vi "BuildCustomDashBoardData.vi"   [LabVIEW 2013]
doc: "This VI builds data and sends it back to the dashboard PC program. By default it sends back the raw values for the first analog, digital, and solenoid module. Modify it to send back the data you want to view. Consider adding higher level data to the Dashboard Datatype.ctl and to this VI. Then update the Dashboard to display the data however you like.\n\nThis software is licensed. Open the labview\\readme\\WPI Robotics Library Open Source License.txt file for more information."
uses:
  <vilib>/Rock Robotics/WPI/DriverStation/WPI_DriverStationDigitalData.ctl
  typedefs/Dashboard Datatype.ctl
  typedefs/DashboardEnable.ctl
  typedefs/custom dash data.ctl
  typedefs/subStates.ctl
  typedefs/vision data.ctl
  <vilib>/Rock Robotics/WPI/Joystick/WPI_JoystickButtonState.ctl
  typedefs/fg_typedef.ctl
  <vilib>/Rock Robotics/SystemInterfaces/System/FPGA_SystemGet.vi
  <vilib>/Rock Robotics/WPI/Joystick/WPI_JoystickGetSetRefNum.vi
  <vilib>/NI_Real-Time Target Support.lvlib
types:
  T1 = typedef "custom dash data.ctl" = cluster{"Motors":cluster{"Pickup Motor":dbl, "Pickup Belt":dbl, "Pickup Distance ":dbl, "Pickup Rate":dbl, "Right Motor":dbl, "Left Motor":dbl}, "substates":cluster{"Latch":T2, "Pickup Arm":T2, "Belts":T2, "Shooter":T2, "Drive":T2}, "Safeties":cluster{"Arm Safety":bool, "Arm Limit":bool}, "Performance":cluster{"CPU Usage":dbl, "Vision mSPI":u32, "Main mSPI":u32}, "Data":T3, "Joysticks":cluster{"J1 Axes":cluster{"axis 1 (x)":dbl, "axis 2 (y)":dbl, "axis 3 (throttle)":dbl, "axis 4":dbl, "axis 5":dbl, "axis 6":dbl}, "J1 Buttons":T4, "J2 Axes":cluster{"axis 1 (x)":dbl, "axis 2 (y)":dbl, "axis 3 (throttle)":dbl, "axis 4":dbl, "axis 5":dbl, "axis 6":dbl}, "J2 Buttons":T4, "J3 Axes":cluster{"axis 1 (x)":dbl, "axis 2 (y)":dbl, "axis 3 (throttle)":dbl, "axis 4":dbl, "axis 5":dbl, "axis 6":dbl}, "J3 Buttons":T4}, "SubSystem Manager":cluster{"Ball State Read":enum16{"no ball", "holding", "loaded"}, "Picked Up":bool, "Loaded":bool, "Shooter Cocked":bool, "Arm Ready":bool}, "Vision Enabled?":bool}
  T2 = typedef "subStates.ctl" = enum16{"null", "wait", "driver control", "auto", "manual override", "hold position", "rotate", "pickup", "pass", "load", "goto shoot", "shoot", "end"}
  T3 = typedef "vision data.ctl" = cluster{"x":dbl, "y":dbl, "area":dbl, "width":dbl, "height":dbl, "Hot Goal Present?":bool, "distance":dbl}
  T4 = typedef "WPI_JoystickButtonState.ctl" = cluster{"Button 1":bool, "Button 2":bool, "Button 3":bool, "Button 4":bool, "Button 5":bool, "Button 6":bool, "Button 7":bool, "Button 8":bool, "Button 9":bool, "Button 10":bool, "Button 11":bool, "Button 12":bool}
  T5 = typedef "DashboardEnable.ctl" = cluster{"Analog Module 1":bool[], "Analog Module 2":bool[], "Digital Module 1":bool, "Digital Module 2":bool, "Solenoid Module":bool}
  T6 = typedef "Dashboard Datatype.ctl" = cluster{cluster{"AnalogModule[0]":cluster{"Channel[0]":sgl, "Channel[1]":sgl, "Channel[2]":sgl, "Channel[3]":sgl, "Channel[4]":sgl, "Channel[5]":sgl, "Channel[6]":sgl, "Channel[7]":sgl}, "AnalogModule[1]":cluster{"Channel[0]":sgl, "Channel[1]":sgl, "Channel[2]":sgl, "Channel[3]":sgl, "Channel[4]":sgl, "Channel[5]":sgl, "Channel[6]":sgl, "Channel[7]":sgl}}, cluster{"DigitalModule[0]":T7, "DigitalModule[1]":T7}, "Solenoid":u8}
  T7 = typedef "WPI_DriverStationDigitalData.ctl" = cluster{"Relay Fwd":u8, "Relay Rev":u8, "GPIO":u16, "GPIO_OE":u16, "PWM":cluster{"PWM[0]":u8, "PWM[1]":u8, "PWM[2]":u8, "PWM[3]":u8, "PWM[4]":u8, "PWM[5]":u8, "PWM[6]":u8, "PWM[7]":u8, "PWM[8]":u8, "PWM[9]":u8}}
  T8 = typedef "fg_typedef.ctl" = enum16{"Get", "Set"}
  T9 = cluster{"AnalogModule[0]":cluster{"Channel[0]":sgl, "Channel[1]":sgl, "Channel[2]":sgl, "Channel[3]":sgl, "Channel[4]":sgl, "Channel[5]":sgl, "Channel[6]":sgl, "Channel[7]":sgl}, "AnalogModule[1]":cluster{"Channel[0]":sgl, "Channel[1]":sgl, "Channel[2]":sgl, "Channel[3]":sgl, "Channel[4]":sgl, "Channel[5]":sgl, "Channel[6]":sgl, "Channel[7]":sgl}}
  T10 = cluster{"DigitalModule[0]":T7, "DigitalModule[1]":T7}
  T11 = cluster{"Channel[0]":sgl, "Channel[1]":sgl, "Channel[2]":sgl, "Channel[3]":sgl, "Channel[4]":sgl, "Channel[5]":sgl, "Channel[6]":sgl, "Channel[7]":sgl}[]
  T12 = cluster{"Channel[0]":sgl, "Channel[1]":sgl, "Channel[2]":sgl, "Channel[3]":sgl, "Channel[4]":sgl, "Channel[5]":sgl, "Channel[6]":sgl, "Channel[7]":sgl}
  T13 = cluster{"AnalogModule[0][0]":sgl, "AnalogModule[0][1]":sgl, "AnalogModule[0][2]":sgl, "AnalogModule[0][3]":sgl, "AnalogModule[0][4]":sgl, "AnalogModule[0][5]":sgl, "AnalogModule[0][6]":sgl, "AnalogModule[0][7]":sgl}
  T14 = cluster{"[0]":cluster{"Channel[0]":sgl, "Channel[1]":sgl, "Channel[2]":sgl, "Channel[3]":sgl, "Channel[4]":sgl, "Channel[5]":sgl, "Channel[6]":sgl, "Channel[7]":sgl}, "[1]":cluster{"Channel[0]":sgl, "Channel[1]":sgl, "Channel[2]":sgl, "Channel[3]":sgl, "Channel[4]":sgl, "Channel[5]":sgl, "Channel[6]":sgl, "Channel[7]":sgl}}
  T15 = typedef "FPGA_DIODevRef.ctl" = cluster{"DevStatus":errorcluster, "Module":T16}
  T16 = typedef "FPGA_TypedefDigitalModule.ctl" = enum16{"Digital Module 1", "Digital Module 2"}
  T17 = cluster{"[0]":u8, "[1]":u8, "[2]":u8, "[3]":u8, "[4]":u8, "[5]":u8, "[6]":u8, "[7]":u8, "[8]":u8, "[9]":u8}
  T18 = typedef "FPGA_SolenoidDevRef.ctl" = cluster{"DevStatus":errorcluster, "Module":T19}
  T19 = typedef "FPGA_TypedefSolenoidModule.ctl" = enum16{"Solenoid Module 1", "Solenoid Module 2"}
  T20 = cluster{"Pickup Motor":dbl, "Pickup Belt":dbl, "Pickup Distance ":dbl, "Pickup Rate":dbl, "Right Motor":dbl, "Left Motor":dbl}
  T21 = cluster{"CPU Usage":dbl, "Vision mSPI":u32, "Main mSPI":u32}
  T22 = typedef "WPI_EncoderDevRef.ctl" = cluster{"DevStatus":errorcluster, "EncoderIndex":T23, "CounterIndex":T24, "DistancePerCount":dbl, "Decoding Type":T25}
  T23 = typedef "FPGA_EncoderIdx.ctl" = enum8{"Enc 0", "Enc 1", "Enc 2", "Enc 3", "Invalid"}
  T24 = typedef "FPGA_CounterCtrSystemIndex.ctl" = enum8{"Ctr 0", "Ctr 1", "Ctr 2", "Ctr 3", "Ctr 4", "Ctr 5", "Ctr 6", "Ctr 7", "Invalid"}
  T25 = typedef "WPI_EncoderType.ctl" = enum16{"1x", "2x", "4x"}
  T26 = typedef "WPI_MotorControlDeviceRef.ctl" = cluster{"DeviceStatus":errorcluster, "Type":enum16{"PWM", "CAN"}, "PWM":cluster{"Digital Module":T16, "PWM Channel":T27, "DeadBand":T28}, "CAN":cluster{"Device Number":u8, "Control Mode":T29, "Semaphore":T30, "Max Vout":dbl}, "Invert":bool, "TransformRef":T31, "InvTransformRef":T31}
  T27 = typedef "FPGA_DIOPWMChannel.ctl" = enum8{"PWM 1", "PWM 2", "PWM 3", "PWM 4", "PWM 5", "PWM 6", "PWM 7", "PWM 8", "PWM 9", "PWM 10", "Invalid"}
  T28 = typedef "WPI_PWMDeadband.ctl" = cluster{"Name":string, "maxPositivePwm":i32, "minPositivePwm":i32, "centerPwm":i32, "maxNegativePwm":i32, "minNegativePwm":i32, "angularRange":u16}
  T29 = typedef "WPI_CANJaguar_ControlMode.ctl" = enum8{"Percent VBus", "Current", "Speed", "Position", "Voltage"}
  T30 = typedef "Semaphore RefNum" = refnum<k1>
  T31 = typedef "WPI_PWMTransform_ConPane.ctl" = refnum<vi>
  T32 = typedef "NI_Real-Time Target Support.lvlib/RT CPU Load.ctl" = cluster{"Total (%)":dbl, "Time Critical (%)":dbl, "Timed Structures (%)":dbl, "High (%)":dbl, "Above Normal (%)":dbl, "Normal (%)":dbl, "Background (%)":dbl, "Idle (%)":dbl, "ISR (%)":dbl}
  T33 = cluster{"Vision mSPI":u32, "Main mSPI":u32, "Dash mSPI":u32}
  T34 = cluster{"Ball State Read":enum16{"no ball", "holding", "loaded"}, "Picked Up":bool, "Loaded":bool, "Shooter Cocked":bool, "Arm Ready":bool}
  T35 = typedef "WPI_JoystickDevRef.ctl" = cluster{"Device":T36}
  T36 = typedef "WPI_JoystickDeviceEnum.ctl" = enum16{"USB 1", "USB 2", "USB 3", "USB 4", "Kinect 1", "Kinect 2"}
  T37 = cluster{"axis 1 (x)":dbl, "axis 2 (y)":dbl, "axis 3 (throttle)":dbl, "axis 4":dbl, "axis 5":dbl, "axis 6":dbl}
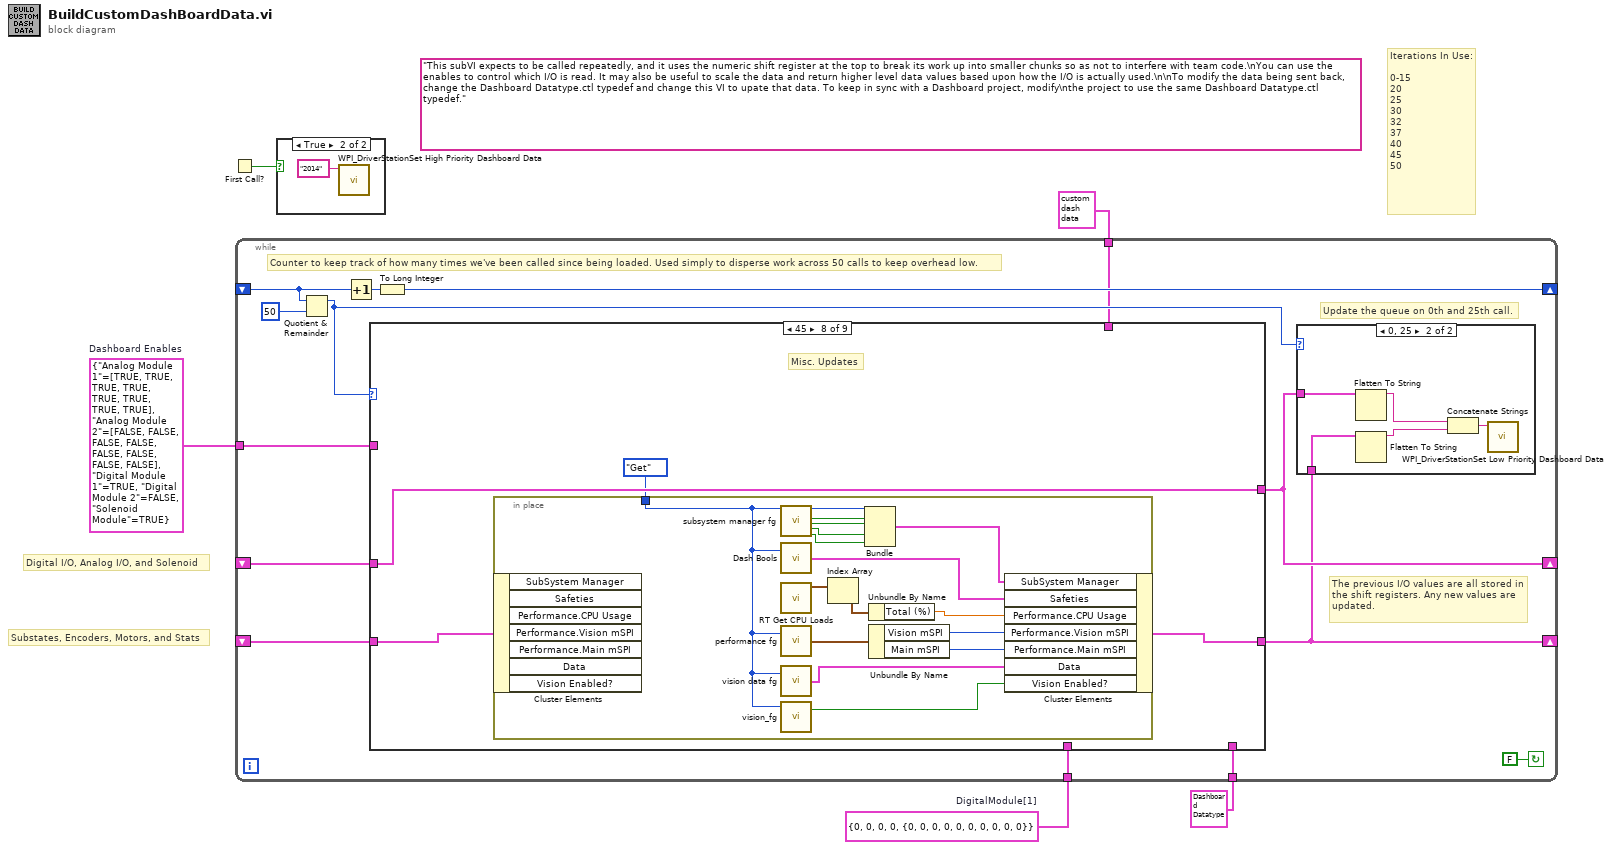
[diagram p0: block diagram]
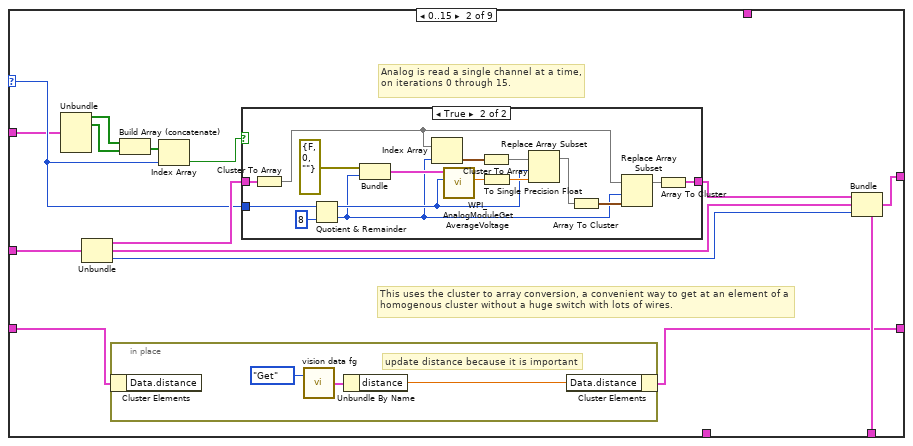
[diagram p5: hidden frame]
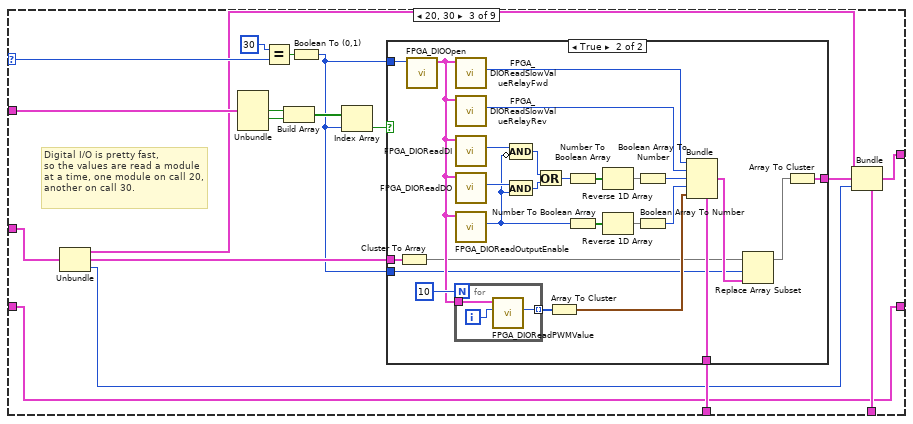
[diagram p7: hidden frame]
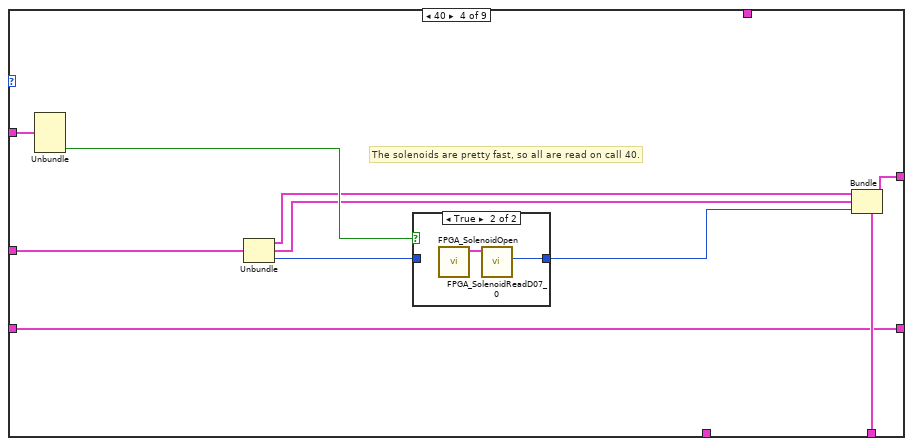
[diagram p9: hidden frame]
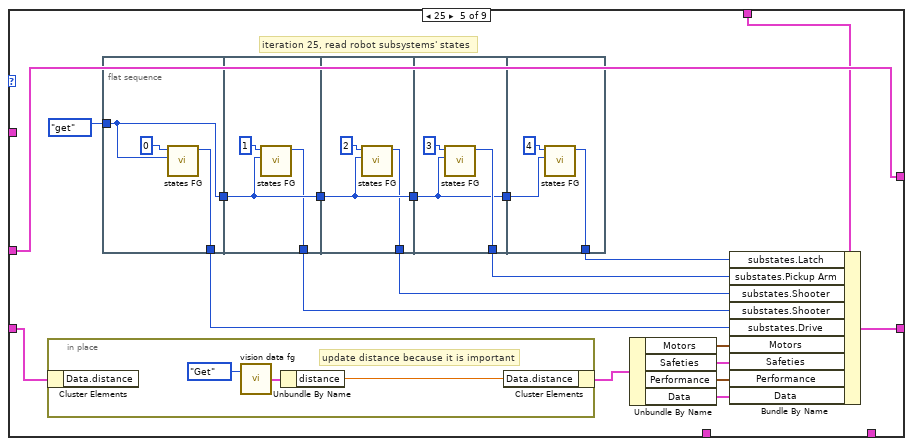
[diagram p11: hidden frame]
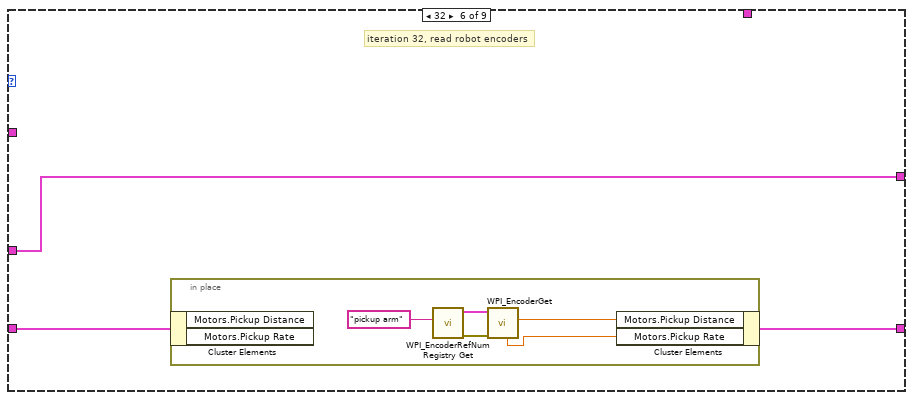
[diagram p12: hidden frame]
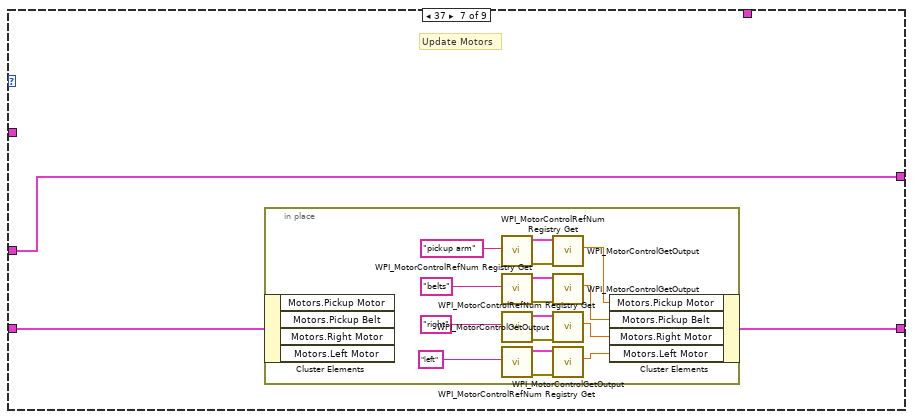
[diagram p13: hidden frame]
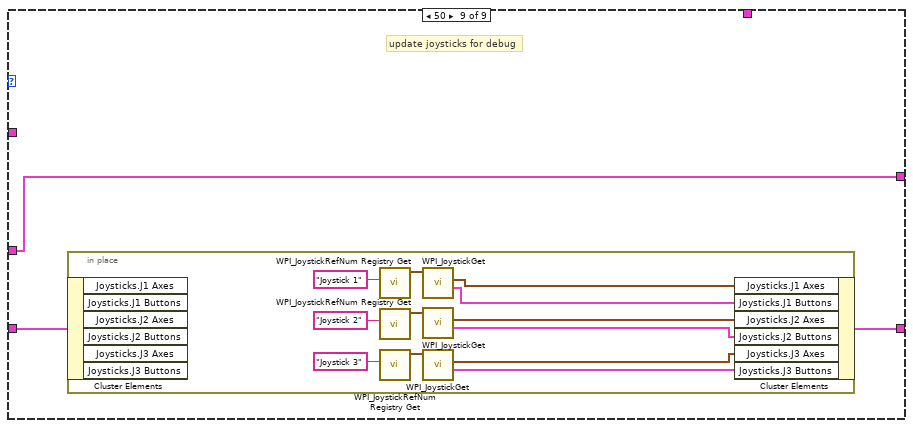
[diagram p14: hidden frame]
diagram:
  w5 = T5 {"Analog Module 1"=[TRUE, TRUE, TRUE, TRUE, TRUE, TRUE, TRUE, TRUE], "Analog Module 2"=[FALSE, FALSE, FALSE, FALSE, FALSE, FALSE, FALSE, FALSE], "Digital Module 1"=TRUE, "Digital Module 2"=FALSE, "Solenoid Module"=TRUE}  # Dashboard Enables
  (unwired) "This subVI expects to be called repeatedly, and it uses the numeric shift register at the top to break its work up into smaller chunks so as not to interfere with team code.\nYou can use the enables to control which I/O is read. It may also be useful to scale the data and return higher level data values based upon how the I/O is actually used.\n\nTo modify the data being sent back, change the Dashboard Datatype.ctl typedef and change this VI to upate that data. To keep in sync with a Dashboard project, modify\nthe project to use the same Dashboard Datatype.ctl typedef."
  w4 = T7 {"Relay Fwd"=0, "Relay Rev"=0, "GPIO"=0, "GPIO_OE"=0, "PWM"={"PWM[0]"=0, "PWM[1]"=0, "PWM[2]"=0, "PWM[3]"=0, "PWM[4]"=0, "PWM[5]"=0, "PWM[6]"=0, "PWM[7]"=0, "PWM[8]"=0, "PWM[9]"=0}}  # DigitalModule[1]
  # "Iterations In Use:\n\n0-15\n20\n25\n30\n32\n37\n40\n45\n50"
  # "Substates, Encoders, Motors, and Stats"
  # "Digital I/O, Analog I/O, and Solenoid"
  n1 = First Call?() -> (First Call?: T/F=w3:bool)
  n2 = while {
    shift-right: [w12] -> _
    shift-left: _ -> [w14]
    shift-right: [w9] -> _
    shift-left: _ -> [w17]
    tunnel: w4 -> [w16]
    tunnel: T6 {{"AnalogModule[0]"={"Channel[0]"=0.0, "Channel[1]"=0.0, "Channel[2]"=0.0, "Channel[3]"=0.0, "Channel[4]"=0.0, "Channel[5]"=0.0, "Channel[6]"=0.0, "Channel[7]"=0.0}, "AnalogModule[1]"={"Channel[0]"=0.0, "Channel[1]"=0.0, "Channel[2]"=0.0, "Channel[3]"=0.0, "Channel[4]"=0.0, "Channel[5]"=0.0, "Channel[6]"=0.0, "Channel[7]"=0.0}}, {"DigitalModule[0]"={"Relay Fwd"=0, "Relay Rev"=0, "GPIO"=0, "GPIO_OE"=0, "PWM"={"PWM[0]"=0, "PWM[1]"=0, "PWM[2]"=0, "PWM[3]"=0, "PWM[4]"=0, "PWM[5]"=0, "PWM[6]"=0, "PWM[7]"=0, "PWM[8]"=0, "PWM[9]"=0}}, "DigitalModule[1]"={"Relay Fwd"=0, "Relay Rev"=0, "GPIO"=0, "GPIO_OE"=0, "PWM"={"PWM[0]"=0, "PWM[1]"=0, "PWM[2]"=0, "PWM[3]"=0, "PWM[4]"=0, "PWM[5]"=0, "PWM[6]"=0, "PWM[7]"=0, "PWM[8]"=0, "PWM[9]"=0}}}, "Solenoid"=0} ("Dashboard Data") -> [w11]
    tunnel: w5 -> [w10]
    shift-right: [w6] -> _
    shift-left: _ -> [w7]
    tunnel: T1 {"Motors"={"Pickup Motor"=0.0, "Pickup Belt"=0.0, "Pickup Distance "=0.0, "Pickup Rate"=0.0, "Right Motor"=0.0, "Left Motor"=0.0}, "substates"={"Latch"=enum."null", "Pickup Arm"=enum."null", "Belts"=enum."null", "Shooter"=enum."null", "Drive"=enum."null"}, "Safeties"={"Arm Safety"=FALSE, "Arm Limit"=FALSE}, "Performance"={"CPU Usage"=0.0, "Vision mSPI"=0, "Main mSPI"=0}, "Data"={"x"=0.0, "y"=0.0, "area"=0.0, "width"=0.0, "height"=0.0, "Hot Goal Present?"=FALSE, "distance"=0.0}, "Joysticks"={"J1 Axes"={"axis 1 (x)"=0.0, "axis 2 (y)"=0.0, "axis 3 (throttle)"=0.0, "axis 4"=0.0, "axis 5"=0.0, "axis 6"=0.0}, "J1 Buttons"={"Button 1"=FALSE, "Button 2"=FALSE, "Button 3"=FALSE, "Button 4"=FALSE, "Button 5"=FALSE, "Button 6"=FALSE, "Button 7"=FALSE, "Button 8"=FALSE, "Button 9"=FALSE, "Button 10"=FALSE, "Button 11"=FALSE, "Button 12"=FALSE}, "J2 Axes"={"axis 1 (x)"=0.0, "axis 2 (y)"=0.0, "axis 3 (throttle)"=0.0, "axis 4"=0.0, "axis 5"=0.0, "axis 6"=0.0}, "J2 Buttons"={"Button 1"=FALSE, "Button 2"=FALSE, "Button 3"=FALSE, "Button 4"=FALSE, "Button 5"=FALSE, "Button 6"=FALSE, "Button 7"=FALSE, "Button 8"=FALSE, "Button 9"=FALSE, "Button 10"=FALSE, "Button 11"=FALSE, "Button 12"=FALSE}, "J3 Axes"={"axis 1 (x)"=0.0, "axis 2 (y)"=0.0, "axis 3 (throttle)"=0.0, "axis 4"=0.0, "axis 5"=0.0, "axis 6"=0.0}, "J3 Buttons"={"Button 1"=FALSE, "Button 2"=FALSE, "Button 3"=FALSE, "Button 4"=FALSE, "Button 5"=FALSE, "Button 6"=FALSE, "Button 7"=FALSE, "Button 8"=FALSE, "Button 9"=FALSE, "Button 10"=FALSE, "Button 11"=FALSE, "Button 12"=FALSE}}, "SubSystem Manager"={"Ball State Read"=enum."no ball", "Picked Up"=FALSE, "Loaded"=FALSE, "Shooter Cocked"=FALSE, "Arm Ready"=FALSE}, "Vision Enabled?"=FALSE} ("Custom Dash Data") -> [w8]
    stop <- FALSE continue-if-true
    # "Counter to keep track of how many times we've been called since being loaded. Used simply to disperse work across 50 calls to keep overhead low."
    # "Update the queue on 0th and 25th call."
    # "The previous I/O values are all stored in\nthe shift registers. Any new values are\nupdated."
    n3 = Quotient & Remainder(x=w14, y=50) -> (x-y*floor(x/y)=w13:i32)  [unwired: 1 out]
    n4 = Increment(x=w14) -> (x+1=w19:i32)
    n5 = case shown="45" w13 {
      selector: w13 -> [_ w36 w75 _ _ _ _ _ _]
      tunnel: [w26 w32 w66 w116 w131 w161 w170 w189 w209] -> w9
      tunnel: w17 -> [w26 w31 w68 w118 w131 w161 w170 w189 w209]
      tunnel: w16 -> [_ _ w79 _ _ _ _ _ _]
      tunnel: w11 -> [_ w38 w67 w115 _ _ _ _ _]
      tunnel: w10 -> [_ w35 w73 w119 _ _ _ _ _]
      tunnel: w8 -> [_ _ _ _ w129 _ _ _ _]
      tunnel: [w25 w27 w64 w112 w130 w162 w169 w190 w207] -> w6
      tunnel: w7 -> [w25 w28 w64 w112 w125 w160 w168 w188 w208]
      frame Default {
        # "Don't update any I/O"
      }
      frame 0..15 {
        # "This uses the cluster to array conversion, a convenient way to get at an element of a\nhomogenous cluster without a huge switch with lots of wires."
        # "Analog is read a single channel at a time,\non iterations 0 through 15."
        n6 = Unbundle(w35) -> ("Analog Module 1"=w34:bool[], "Analog Module 2"=w33:bool[])  [unwired: 3 out]
        n7 = Unbundle(w31) -> (w37:T9, w30:T10, "Solenoid"=w29:u8)
        n8 = in-place {
          # "update distance because it is important"
          n9 = in-place-cluster #1(w28) -> ()  [unwired: 1 out]
          n10 = call "vision data fg.vi"("Menu"=fg_typedef."Get") -> ("Output"=w43:T3)  [unwired: 1 in]
          n11 = Unbundle By Name(w43) -> ("distance"=w42:dbl)
          n12 = in-place-cluster #1("Data.distance"=w42) -> (w27:T1)
        }
        n13 = Build Array (concatenate)(w34, w33) -> (w40:bool[])
        n14 = Index Array(array=w40, index=w36) -> (element=w41:bool)
        n15 = case shown="True" w41 {
          tunnel: w36 -> [_ w52]
          tunnel: [w45 w49] -> w39
          tunnel: w37 -> [w45 w48]
          frame False {
          }
          frame True {
            n16 = Cluster To Array(cluster=w48) -> (array=w47:T11)
            n17 = Quotient & Remainder(x=w52, y=8) -> (x-y*floor(x/y)=w51:i32, floor(x/y)=w46:i32)
            n18 = Bundle("DevStatus"=errorcluster {"status"=FALSE, "code"=0, "source"=""}, w46) -> (w60:cluster{"DevStatus":errorcluster, i32})  [unwired: 1 out]
            n19 = Index Array(array=w47, index=w46) -> (element=w54:T12)
            n20 = call <vilib>:"WPI_AnalogModuleGetAverageVoltage.vi"("Channel"=w51, "AnalogModuleDevStatus"=w60) -> ("Average Voltage"=w57:dbl)  [unwired: 1 in, 8 out]
            n21 = Cluster To Array(cluster=w54) -> (array=w53:sgl[])
            n22 = To Single Precision Float(number=w57) -> (single precision float=w56:sgl)
            n23 = Replace Array Subset(array=w53, new element=w56, index=w51) -> (w55:sgl[])
            n24 = Array To Cluster(array=w55) -> (cluster=w59:T13)
            n25 = Replace Array Subset(array=w47, new element=w59, index=w46) -> (w50:T11)
            n26 = Array To Cluster(array=w50) -> (cluster=w49:T14)
          }
        }
        n27 = Bundle(cluster=w38, w39, w30, "Solenoid"=w29) -> (w32:T6)
      }
      frame 20, 30 {
        # "Digital I/O is pretty fast,\nso the values are read a module\nat a time, one module on call 20,\nanother on call 30."
        n28 = Unbundle(w68) -> (w63:T9, w70:T10, "Solenoid"=w62:u8)
        n29 = Unbundle(w73) -> ("Digital Module 1"=w72:bool, "Digital Module 2"=w71:bool)  [unwired: 3 out]
        n30 = Equal?(x=30, y=w75) -> (x = y?=w77:bool)
        n31 = Build Array(w72, w71) -> (w74:bool[])
        n32 = Boolean To (0,1)(Boolean=w77) -> (0, 1=w65:i16)
        n33 = Index Array(array=w74, index=w65) -> (element=w76:bool)
        n34 = case shown="True" w76 {
          tunnel: w79 -> [_ w88]
          tunnel: [w80 w81] -> w69
          tunnel: w65 -> [_ w86]
          tunnel: w65 -> [_ w85]
          tunnel: w70 -> [w80 w84]
          frame False {
          }
          frame True {
            n35 = Cluster To Array(cluster=w84) -> (array=w83:T7[])
            n36 = call <vilib>:"FPGA_DIOOpen.vi"("Module (Module 1)"=w86) -> ("DIODeviceRef"=w104:T15)  [unwired: 1 in, 9 out]
            n37 = for {
              N: 10 -> [_]
              tunnel: w104 -> [w109]
              tunnel: [w107] -> w105 mode=indexing
              i -> [w108]
              n38 = call <vilib>:"FPGA_DIOReadPWMValue.vi"("PWMChannel"=w108, "DIODeviceRef In"=w109) -> ("PWMValue"=w107:u8)  [unwired: 1 in, 8 out]
            }
            n39 = call <vilib>:"FPGA_DIOReadSlowValueRelayFwd.vi"("DIODeviceRef In"=w104) -> ("Relay Forward"=w97:u8)  [unwired: 1 in, 9 out]
            n40 = call <vilib>:"FPGA_DIOReadSlowValueRelayRev.vi"("DIODeviceRef In"=w104) -> ("Relay Reverse"=w98:u8)  [unwired: 1 in, 9 out]
            n41 = call <vilib>:"FPGA_DIOReadDI.vi"("DIODeviceRef In"=w104) -> ("DI"=w102:u16)  [unwired: 1 in, 9 out]
            n42 = call <vilib>:"FPGA_DIOReadDO.vi"("DIODeviceRef In"=w104) -> ("DO"=w101:u16)  [unwired: 1 in, 9 out]
            n43 = call <vilib>:"FPGA_DIOReadOutputEnable.vi"("DIODeviceRef In"=w104) -> ("OutputEnable"=w92:u16)  [unwired: 1 in, 9 out]
            n44 = And(x=w101, y=w92) -> (x .and. y?=w100:u16)
            n45 = Compound Arithmetic op=AND(w102, invert w92) -> (w99:u16)
            n46 = Or(x=w99, y=w100) -> (x .or. y?=w90:u16)
            n47 = Array To Cluster(array=w105) -> (cluster=w103:T17)
            n48 = Number To Boolean Array(number=w90) -> (Boolean array=w95:bool[])
            n49 = Number To Boolean Array(number=w92) -> (Boolean array=w94:bool[])
            n50 = Reverse 1D Array(array=w95) -> (reversed array=w96:bool[])
            n51 = Reverse 1D Array(array=w94) -> (reversed array=w93:bool[])
            n52 = Boolean Array To Number(Boolean array=w96) -> (number=w89:u32)
            n53 = Boolean Array To Number(Boolean array=w93) -> (number=w91:u32)
            n54 = Bundle(cluster=w88, "Relay Fwd"=w97, "Relay Rev"=w98, "GPIO"=w89, "GPIO_OE"=w91, "PWM"=w103) -> (w87:T7)
            n55 = Replace Array Subset(array=w83, new element=w87, index=w85) -> (w82:T7[])
            n56 = Array To Cluster(array=w82) -> (cluster=w81:cluster{"[0]":T7, "[1]":T7})
          }
        }
        n57 = Bundle(cluster=w67, w63, w69, "Solenoid"=w62) -> (w66:T6)
      }
      frame 40 {
        # "The solenoids are pretty fast, so all are read on call 40."
        n58 = Unbundle(w119) -> ("Solenoid Module"=w113:bool)  [unwired: 4 out]
        n59 = Unbundle(w118) -> (w111:T9, w110:T10, "Solenoid"=w117:u8)
        n60 = case shown="True" w113 {
          tunnel: [w120 w121] -> w114
          tunnel: w117 -> [w120 _]
          frame False {
          }
          frame True {
            n61 = call <vilib>:"FPGA_SolenoidOpen.vi"() -> ("SolenoidDevRef"=w122:T18)  [unwired: 2 in, 9 out]
            n62 = call <vilib>:"FPGA_SolenoidReadD07_0.vi"("SolenoidDevRef"=w122) -> ("DO7:0"=w121:u8)  [unwired: 1 in, 9 out]
          }
        }
        n63 = Bundle(cluster=w115, w111, w110, "Solenoid"=w114) -> (w116:T6)
      }
      frame 25 {
        # "iteration 25, read robot subsystems' states"
        n64 = in-place {
          # "update distance because it is important"
          n65 = in-place-cluster #2(w125) -> ()  [unwired: 1 out]
          n66 = call "vision data fg.vi"("Menu"=fg_typedef."Get") -> ("Output"=w143:T3)  [unwired: 1 in]
          n67 = Unbundle By Name(w143) -> ("distance"=w142:dbl)
          n68 = in-place-cluster #2("Data.distance"=w142) -> (w124:T1)
        }
        n69 = flat-sequence {
          tunnel: enum16{"set", "get"}."get" ("menu (get)") -> [w147]
          tunnel: [w147] -> w138
          tunnel: [w145] -> w132
          tunnel: [w150] -> w139
          tunnel: w138 -> [w150]
          tunnel: [w148] -> w133
          tunnel: [w153] -> w140
          tunnel: w139 -> [w153]
          tunnel: [w151] -> w134
          tunnel: w140 -> [w154]
          tunnel: [w155] -> w135
          tunnel: [w154] -> w137
          tunnel: w137 -> [w158]
          tunnel: [w157] -> w136
          frame #0 {
            n70 = call "states FG.vi"("menu (get)"=w147, "Loop ID"=0) -> ("subState out"=w145:T2)  [unwired: 6 in, 3 out]
          }
          frame #1 {
            n71 = call "states FG.vi"("menu (get)"=w150, "Loop ID"=1) -> ("subState out"=w148:T2)  [unwired: 6 in, 3 out]
          }
          frame #2 {
            n72 = call "states FG.vi"("menu (get)"=w153, "Loop ID"=2) -> ("subState out"=w151:T2)  [unwired: 6 in, 3 out]
          }
          frame #3 {
            n73 = call "states FG.vi"("menu (get)"=w154, "Loop ID"=3) -> ("subState out"=w155:T2)  [unwired: 6 in, 3 out]
          }
          frame #4 {
            n74 = call "states FG.vi"("menu (get)"=w158, "Loop ID"=4) -> ("subState out"=w157:T2)  [unwired: 6 in, 3 out]
          }
        }
        n75 = Unbundle By Name(w124) -> ("Motors"=w123:T20, "Safeties"=w128:cluster{"Arm Safety":bool, "Arm Limit":bool}, "Performance"=w127:T21, "Data"=w126:T3)
        n76 = Bundle By Name(cluster=w129, "substates.Latch"=w136, "substates.Pickup Arm"=w135, "substates.Shooter"=w134, "substates.Shooter"=w133, "substates.Drive"=w132, "Motors"=w123, "Safeties"=w128, "Performance"=w127, "Data"=w126) -> (w130:T1)
      }
      frame 32 {
        # "iteration 32, read robot encoders"
        n77 = in-place {
          n78 = in-place-cluster #3(w160) -> ()  [unwired: 2 out]
          n79 = call <vilib>:"WPI_EncoderRefNum Registry Get.vi"("refnum name"="pickup arm") -> ("error out"=w166:errorcluster, "EncoderDevRef"=w167:T22)  [unwired: 9 in]
          n80 = call <vilib>:"WPI_EncoderGet.vi"("error in (no error)"=w166, "EncoderDevRef"=w167) -> ("Distance"=w164:dbl, "Rate"=w163:dbl)  [unwired: 4 in, 4 out]
          n81 = in-place-cluster #3("Motors.Pickup Distance"=w164, "Motors.Pickup Rate"=w163) -> (w162:T1)
        }
      }
      frame 37 {
        # "Update Motors"
        n82 = in-place {
          n83 = in-place-cluster #4(w168) -> ()  [unwired: 4 out]
          n84 = call <vilib>:"WPI_MotorControlRefNum Registry Get.vi"("refnum name"="pickup arm") -> ("error out"=w179:errorcluster, "MotorControlDevRef"=w183:T26)  [unwired: 9 in]
          n85 = call <vilib>:"WPI_MotorControlRefNum Registry Get.vi"("refnum name"="belts") -> ("error out"=w180:errorcluster, "MotorControlDevRef"=w186:T26)  [unwired: 9 in]
          n86 = call <vilib>:"WPI_MotorControlRefNum Registry Get.vi"("refnum name"="right") -> ("error out"=w178:errorcluster, "MotorControlDevRef"=w176:T26)  [unwired: 9 in]
          n87 = call <vilib>:"WPI_MotorControlRefNum Registry Get.vi"("refnum name"="left") -> ("error out"=w173:errorcluster, "MotorControlDevRef"=w175:T26)  [unwired: 9 in]
          n88 = call <vilib>:"WPI_MotorControlGetOutput.vi"("error in (no error)"=w179, "MotorControlDevRef"=w183) -> ("Output"=w182:dbl)  [unwired: 7 in, 2 out]
          n89 = call <vilib>:"WPI_MotorControlGetOutput.vi"("error in (no error)"=w180, "MotorControlDevRef"=w186) -> ("Output"=w181:dbl)  [unwired: 7 in, 2 out]
          n90 = call <vilib>:"WPI_MotorControlGetOutput.vi"("error in (no error)"=w178, "MotorControlDevRef"=w176) -> ("Output"=w171:dbl)  [unwired: 7 in, 2 out]
          n91 = call <vilib>:"WPI_MotorControlGetOutput.vi"("error in (no error)"=w173, "MotorControlDevRef"=w175) -> ("Output"=w172:dbl)  [unwired: 7 in, 2 out]
          n92 = in-place-cluster #4("Motors.Pickup Motor"=w182, "Motors.Pickup Belt"=w181, "Motors.Right Motor"=w171, "Motors.Left Motor"=w172) -> (w169:T1)
        }
      }
      frame 45 {
        # "Misc. Updates"
        n93 = in-place {
          in-place-border: fg_typedef."Get" ("Menu (Get)") -> [w192]
          n94 = in-place-cluster #5(w188) -> ()  [unwired: 7 out]
          n95 = call "subsystem manager fg.vi"("Menu"=w192) -> ("Ball State Read"=w198:enum16{"no ball", "holding", "loaded"}, "Picked Up"=w197:bool, "Loaded"=w196:bool, "Shooter Cocked"=w195:bool, "Arm Ready"=w194:bool)  [unwired: 14 in]
          n96 = call "Dash Bools.vi"("Menu"=w192) -> ("Output"=w200:cluster{"Arm Safety":bool, "Arm Limit":bool})  [unwired: 1 in]
          n97 = call <vilib>:"RT Get CPU Loads.vi"() -> ("CPU loads"=w205:T32[])  [unwired: 10 in, 1 out]
          n98 = call "performance fg.vi"("Menu"=w192) -> ("Output"=w201:T33)  [unwired: 1 in]
          n99 = call "vision data fg.vi"("Menu"=w192) -> ("Output"=w199:T3)  [unwired: 1 in]
          n100 = call "vision_fg.vi"("Menu"=w192) -> ("Enabled?"=w191:bool)  [unwired: 2 in, 1 out]
          n101 = Index Array(array=w205) -> (element=w206:T32)  [unwired: 1 in]
          n102 = Bundle("Ball State Read"=w198, "Picked Up"=w197, "Loaded"=w196, "Shooter Cocked"=w195, "Arm Ready"=w194) -> (w193:T34)  [unwired: 1 in]
          n103 = Unbundle By Name(w206) -> ("Total (%)"=w204:dbl)
          n104 = Unbundle By Name(w201) -> ("Vision mSPI"=w203:u32, "Main mSPI"=w202:u32)
          n105 = in-place-cluster #5("SubSystem Manager"=w193, "Safeties"=w200, "Performance.CPU Usage"=w204, "Performance.Vision mSPI"=w203, "Performance.Main mSPI"=w202, "Data"=w199, "Vision Enabled?"=w191) -> (w190:T1)
        }
      }
      frame 50 {
        # "update joysticks for debug"
        n106 = in-place {
          n107 = in-place-cluster #6(w208) -> ()  [unwired: 6 out]
          n108 = call <vilib>:"WPI_JoystickRefNum Registry Get.vi"("refnum name"="Joystick 1") -> ("JoystickDevRef"=w218:T35)  [unwired: 9 in, 1 out]
          n109 = call <vilib>:"WPI_JoystickRefNum Registry Get.vi"("refnum name"="Joystick 2") -> ("JoystickDevRef"=w217:T35)  [unwired: 9 in, 1 out]
          n110 = call <vilib>:"WPI_JoystickRefNum Registry Get.vi"("refnum name"="Joystick 3") -> ("JoystickDevRef"=w216:T35)  [unwired: 9 in, 1 out]
          n111 = call <vilib>:"WPI_JoystickGet.vi"("JoystickDevRef"=w218) -> ("Buttons"=w211:T4, "Axes"=w210:T37)  [unwired: 4 in, 1 out]
          n112 = call <vilib>:"WPI_JoystickGet.vi"("JoystickDevRef"=w217) -> ("Buttons"=w213:T4, "Axes"=w212:T37)  [unwired: 4 in, 1 out]
          n113 = call <vilib>:"WPI_JoystickGet.vi"("JoystickDevRef"=w216) -> ("Buttons"=w214:T4, "Axes"=w215:T37)  [unwired: 4 in, 1 out]
          n114 = in-place-cluster #6("Joysticks.J1 Axes"=w210, "Joysticks.J1 Buttons"=w211, "Joysticks.J2 Axes"=w212, "Joysticks.J2 Buttons"=w213, "Joysticks.J3 Axes"=w215, "Joysticks.J3 Buttons"=w214) -> (w207:T1)
        }
      }
    }
    n115 = To Long Integer(number=w19) -> (32bit integer=w12:i32)
    n116 = case shown="0, 25" w13 {
      tunnel: w9 -> [_ w24]
      tunnel: w6 -> [_ w22]
      frame Default {
      }
      frame 0, 25 {
        n117 = Flatten To String(anything=w24) -> (data string=w23:string)  [unwired: 1 in, 4 out]
        n118 = Flatten To String(anything=w22) -> (data string=w20:string)  [unwired: 1 in, 4 out]
        n119 = Concatenate Strings(w23, w20) -> (w21:string)
        n120 = call <vilib>:"WPI_DriverStationSet Low Priority Dashboard Data.vi"("User Data"=w21) -> ()  [unwired: 1 in, 10 out]
      }
    }
  }
  n121 = case shown="True" w3 {
    frame False {
    }
    frame True {
      n122 = call <vilib>:"WPI_DriverStationSet High Priority Dashboard Data.vi"("User Data"="2014") -> ()  [unwired: 10 in, 1 out]
    }
  }
